vi "Alias Already Exists Error.vi"() -> (2 "Error":errorcluster)   [LabVIEW 2021, in "jettl.lvlib"]
uses:
  jettl.lvlib
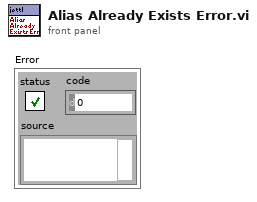
[diagram p1: front panel]
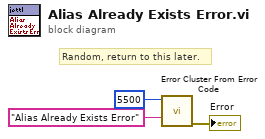
[diagram p0: block diagram]
diagram:
  # "Random, return to this later."
  n1 = call <vilib>:"Error Cluster From Error Code.vi"("error message (\"\")"="Alias Already Exists Error" ("error message (\"\")"), "error code (0)"=5500) -> ("error out"=→"Error":errorcluster)  [unwired: 7 in]
